vi "Pi_BuildBinaryArray.vi"(10 "String in":string) -> (2 "Binary String out":string)   [LabVIEW 2019]
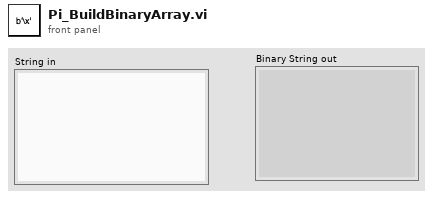
[diagram p1: front panel]
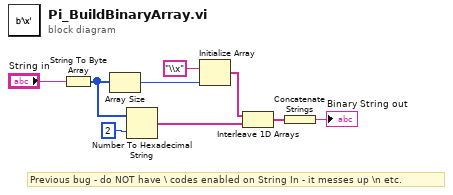
[diagram p0: block diagram]
diagram:
  # "Previous bug - do NOT have \\ codes enabled on String In - it messes up \\n etc."
  n1 = String To Byte Array(string="String in") -> (unsigned byte array=w6:u8[])
  n2 = Array Size(array=w6) -> (size(s)=w5:i32)
  n3 = Number To Hexadecimal String(1:i16 2 ("width (-)"), 2:w6) -> (0:w7:string[])
  n4 = Initialize Array("\\x", w5) -> (w3:string[])
  n5 = Interleave 1D Arrays(w3, w7) -> (w1:string[])
  n6 = Concatenate Strings(w1) -> (→"Binary String out":string)
